vi "ProdaNG.Language.Set.vi"(8 "error in":errorcluster, 10 "languageId (0: English)":i32, 11 "dbHandleIn":i32) -> (0 "error out":errorcluster, 3 "dbHandle":i32)   [LabVIEW 2016]
doc: "This function sets the wanted language for this session and overwrites the default value respective Preference LANGUAGEID with it.\nIn subsequent functions, that delivers or writes language-dependent data, the id specifies language that should be used. If a description is not existent in the desired language, the description is taken from the language 0 (English).\nIf a language-dependent description is inserted or changed, it is being marked with the currently set language. Additionally this description is deposited for language 0, in case that the description does not exist and the current language is not 0.\nParameter:\nhandle is an Integer, that is returned by the function Login() when a new connection is created.\nlanguageId is the Id of one language, which is returned from GetLanguages().\n\nReturncodes:\n0 No error\n< 0 ORACLE error code\n6 (ERROR_INVALID_HANDLE) in case of an invalid handle\n232 (ERROR_NO_DATA) in case of an invalid Id."
uses:
  prodllNG.dll
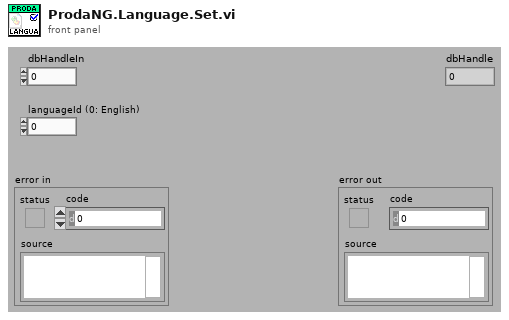
[diagram p1: front panel]
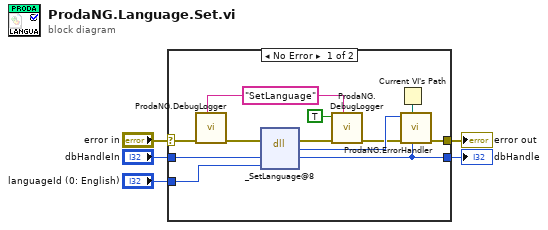
[diagram p0: block diagram]
diagram:
  n1 = case shown="No Error" "error in" {
    selector: "error in" -> [w13 w19]
    tunnel: [w17 w19] -> w4
    tunnel: "dbHandleIn" -> [w16 w18]
    tunnel: "languageId (0: English)" -> [w8 _]
    tunnel: [w7 w18] -> w1
    frame No Error {
      w15 = "SetLanguage" ("cmd")
      n2 = call "ProdaNG.DebugLogger.vi"("cmd"=w15, "error in (no error)"=w13) -> ("error out"=w12:errorcluster)  [unwired: 9 in]
      n3 = dll-call lib="D:/Maszup/WABCO/SVN/LineTraceSystem/SOFTWARE/sources/Database/ProdaNG/prodllNG.dll" fn="_SetLanguage@8" ("ProDll.dll:Login")(error in=w12, "dbHandle"=w16, "languageId"=w8) -> (error out=w11:errorcluster, w10:i32, "dbHandle"=w7:i32)  [unwired: 3 in, 1 out]
      n4 = call "ProdaNG.DebugLogger.vi"("cmd"=w15, "error in (no error)"=w11, "done? (F)"=TRUE) -> ("error out"=w6:errorcluster)  [unwired: 8 in]
      n5 = Current VI's Path() -> (path=w9:path)
      n6 = call "ProdaNG.ErrorHandler.vi"("dbHandleIn"=w7, "Path"=w9, "error in"=w6, "output_parameter"=w10) -> ("error out"=w17:errorcluster)  [unwired: 7 in]
    }
    frame Error {
    }
  }
  "error out" <- w4
  "dbHandle" <- w1
